vi "SetVolume.vi"(0 "reference in":refnum<class "MusicSystem.lvclass">, 2 "RoomName":string, 3 "Volume":u8, 5 "Error In":errorcluster) -> (14 "reference out":refnum<class "MusicSystem.lvclass">, 19 "Error Out":errorcluster)   [LabVIEW 2024, in "MusicSystem.lvclass"]
uses:
  MusicSystem.lvclass
  House/Room_class/Room.lvclass
  Devices/MusicDevice_class/MusicDevice.lvclass
  MusicSystem.lvclass/MusicSystem.ctl
panel:
  # "Connector Pane"
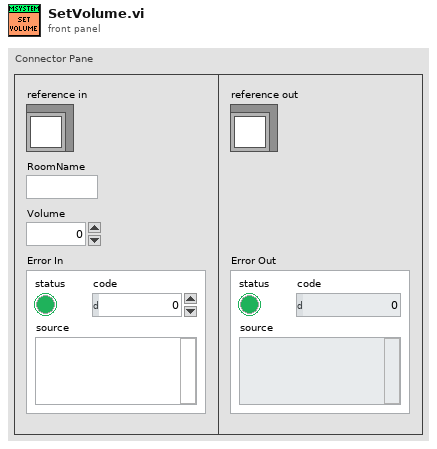
[diagram p1: front panel]
types:
  T1 = typedef "MusicSystem.lvclass/ObjectAttributes.ctl" = cluster{"Rooms":T2}
  T2 = typedef "Rooms Map.ctl" = map{string, refnum<class "Room.lvclass">}
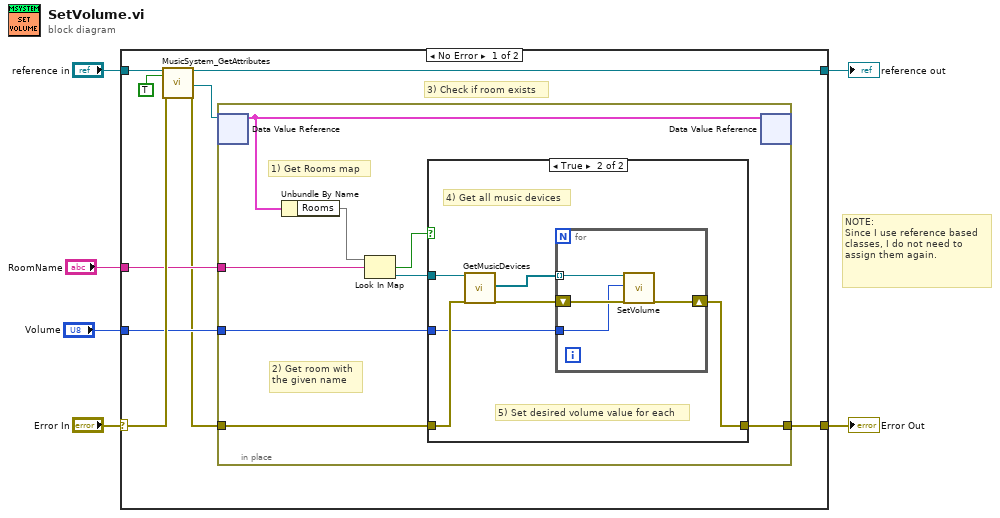
[diagram p0: block diagram]
diagram:
  # "NOTE:\nSince I use reference based classes, I do not need to\nassign them again."
  n1 = case shown="No Error" "Error In" {
    selector: "Error In" -> [w14 w36]
    tunnel: [w7 w36] -> w5
    tunnel: [w13 w35] -> w3
    tunnel: "reference in" -> [w15 w35]
    tunnel: "RoomName" -> [w10 _]
    tunnel: "Volume" -> [w9 _]
    frame No Error {
      # "3) Check if room exists"
      n2 = call "MusicSystem_GetAttributes.vi"("reference in"=w15, "OnlyGetDvrReference(False)"=TRUE, "Error In"=w14) -> ("reference out"=w13:refnum<class "MusicSystem.lvclass">, "DataRef"=w11:refnum<data-value>, "Error Out"=w8:errorcluster)  [unwired: 13 in, 1 out]
      n3 = in-place {
        in-place-border: w10 -> [w21]
        in-place-border: w8 -> [w18]
        in-place-border: [w17] -> w7
        in-place-border: w9 -> [w16]
        # "1) Get Rooms map"
        # "2) Get room with\nthe given name"
        n4 = in-place-dvr #1(w11) -> (w23:T1)  [unwired: 1 out]
        n5 = Unbundle By Name(w23) -> ("Rooms"=w22:T2)
        n6 = Look In Map(map=w22, key=w21) -> (key not found?=w20:bool, value=w19:refnum<class "Room.lvclass">)  [unwired: 1 in]
        n7 = case shown="True" w20 {
          tunnel: w19 -> [_ w30]
          tunnel: w18 -> [w24 w27]
          tunnel: [w24 w26] -> w17
          tunnel: w16 -> [_ w25]
          frame False {
          }
          frame True {
            # "5) Set desired volume value for each"
            # "4) Get all music devices"
            n8 = call-dynamic "GetMusicDevices.vi"("reference in"=w30, "Error In"=w27) -> ("MusicDevices"=w28:refnum<class "MusicDevice.lvclass">[], "Error Out"=w29:errorcluster)  [unwired: 15 in, 1 out]
            n9 = for {
              tunnel: w28 -> [w33] mode=indexing
              shift-right: [w32] -> w26
              shift-left: w29 -> [w34]
              tunnel: w25 -> [w31]
              n10 = call-dynamic "SetVolume.vi"("reference in"=w33, "Volume"=w31, "Error In"=w34) -> ("Error Out"=w32:errorcluster)  [unwired: 15 in, 1 out]
            }
          }
        }
        n11 = in-place-dvr #1(w23) -> ()  [unwired: 2 out]
      }
    }
    frame Error {
    }
  }
  "Error Out" <- w5
  "reference out" <- w3
